vi "Process_day_file.vi"(2 "Filename":path=path "/G3_3 HD/EnFlo Data/Oct_2000/3_Oct") -> (6 "Day KW Hrs":dbl, 7 "Night KWHrs":dbl format="%.2f", 10 "Time":dbl)   [LabVIEW 2010]
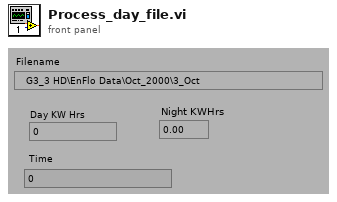
[diagram p1: front panel]
types:
  T1 = cluster{"second":i32, "minute":i32, "hour":i32, "day of month":i32, "month":i32, "year":i32, "day of week":i32, "day of year":i32, "is DST":i32}
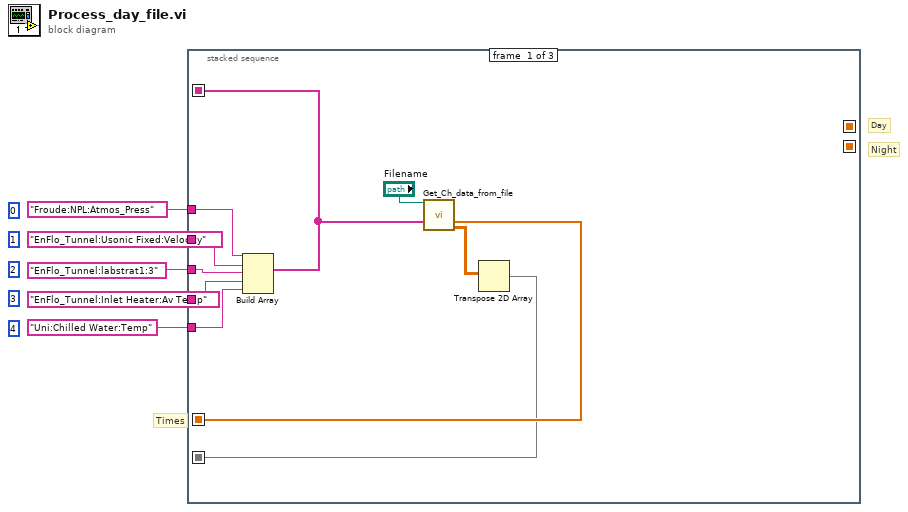
[diagram p0: block diagram]
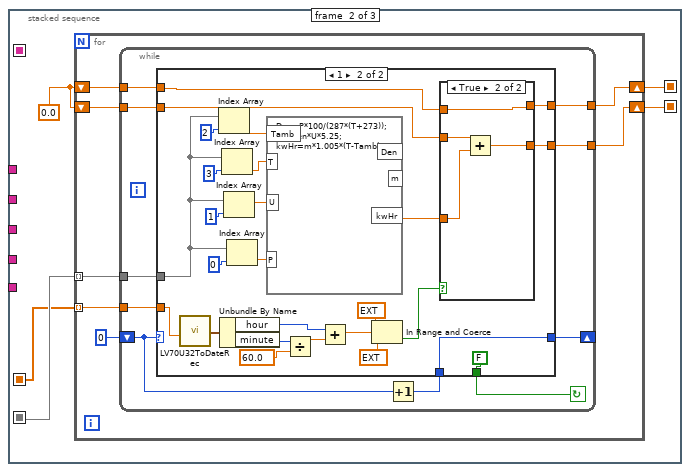
[diagram p2: hidden frame]
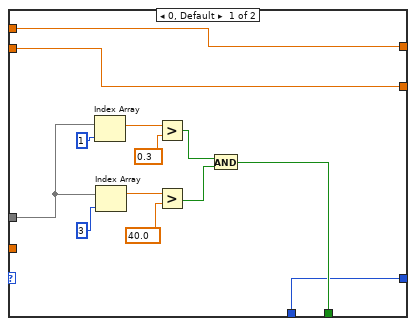
[diagram p3: hidden frame]
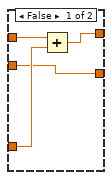
[diagram p4: hidden frame]
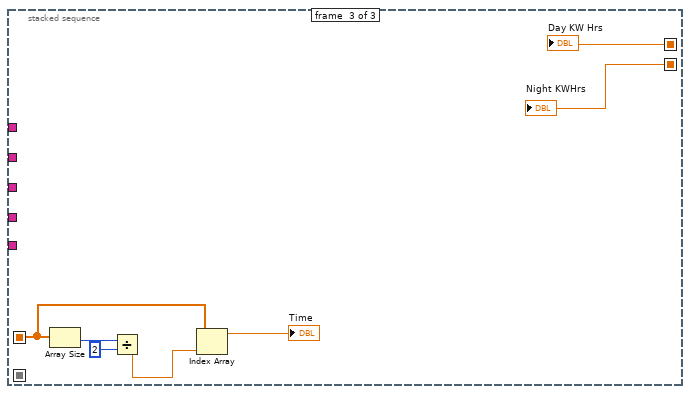
[diagram p5: hidden frame]
diagram:
  (unwired) 4
  (unwired) 3
  (unwired) 2
  (unwired) 1
  (unwired) 0
  # "Night"
  # "Day"
  # "Times"
  n1 = stacked-sequence {
    seq-local: [w9 _ _] -> [_ _ _]
    seq-local: [w8 _ _] -> [_ w18 w87]
    seq-local: [w6 _ _] -> [_ w20 _]
    seq-local: [_ w19 _] -> [_ _ w91]
    seq-local: [_ w16 _] -> [_ _ w85]
    tunnel: "Froude:NPL:Atmos_Press" -> [w15 _ _]
    tunnel: "EnFlo_Tunnel:Usonic Fixed:Velocity" -> [w14 _ _]
    tunnel: "EnFlo_Tunnel:labstrat1:3" -> [w13 _ _]
    tunnel: "EnFlo_Tunnel:Inlet Heater:Av Temp" -> [w12 _ _]
    tunnel: "Uni:Chilled Water:Temp" -> [w11 _ _]
    frame #0 {
      n2 = Build Array(w15, w14, w13, w12, w11) -> (w9:string[])
      n3 = call "Get_Ch_data_from_file.vi"("Filename"="Filename", "Channel names"=w9) -> ("Times"=w8:dbl[], "Ch Data"=w7:dbl[][])  [unwired: 2 in, 10 out]
      n4 = Transpose 2D Array(2D array=w7) -> (transposed array=w6:dbl[][])
    }
    frame #1 {
      w17 = 0.0
      n5 = for {
        tunnel: w20 -> [w26] mode=indexing
        shift-right: [w25] -> w19
        shift-left: w17 -> [w24]
        shift-right: [w21] -> w16
        shift-left: w17 -> [w22]
        tunnel: w18 -> [w23] mode=indexing
        n6 = while {
          tunnel: [w28] -> w21
          tunnel: w22 -> [w29]
          tunnel: w23 -> [w30]
          tunnel: w24 -> [w31]
          tunnel: [w32] -> w25
          tunnel: w26 -> [w37]
          shift-left: 0 -> [w35]
          shift-right: [w33] -> _
          stop <- w36 continue-if-true
          n7 = Increment(x=w35) -> (x+1=w34:i32)
          n8 = case shown="1" w35 {
            tunnel: w37 -> [w46 w72]
            tunnel: [w41 FALSE] -> w36
            tunnel: w34 -> [w40 w63]
            tunnel: [w40 w63] -> w33
            tunnel: [w39 w65] -> w32
            tunnel: w31 -> [w39 w66]
            tunnel: w30 -> [_ w62]
            tunnel: w29 -> [w38 w57]
            tunnel: [w38 w56] -> w28
            frame 0, Default {
              n9 = Index Array(array=w46, index=1 ("Index")) -> (element=w45:dbl)
              n10 = Index Array(array=w46, index=3 ("Index")) -> (element=w49:dbl)
              n11 = Greater?(x=w45, y=0.3) -> (0:w42:bool)
              n12 = Greater?(x=w49, y=40.0) -> (0:w43:bool)
              n13 = And(x=w42, y=w43) -> (x .and. y?=w41:bool)
            }
            frame 1 {
              n14 = call <vilib>:"LV70U32ToDateRec.vi"("Time"=w62) -> ("date time rec"=w61:T1)
              n15 = Index Array(array=w72, index=2 ("Index")) -> (element=w68:dbl)
              n16 = Unbundle By Name(w61) -> ("hour"=w52:i32, "minute"=w55:i32)
              n17 = Index Array(array=w72, index=3 ("Index")) -> (element=w69:dbl)
              n18 = Index Array(array=w72, index=1 ("Index")) -> (element=w70:dbl)
              n19 = Index Array(array=w72, index=0 ("Index")) -> (element=w71:dbl)
              n20 = formula code="Den=P*100/(287*(T+273));\nm=Den*U*5.25;\nkwHr=m*1.005*(T-Tamb)/30;"("Tamb"=w68, "T"=w69, "U"=w70, "P"=w71) -> ("kwHr"=w67:dbl)  [unwired: 2 out]
              n21 = Divide(x=w55, y=60.0) -> (x/y=w53:dbl)
              n22 = Add(x=w52, y=w53) -> (x+y=w51:dbl)
              n23 = In Range and Coerce(upper limit=ext 7.5 ("hi"), x=w51, lower limit=ext 0.5 ("lo")) -> (In Range?=w58:bool)  [unwired: 1 out]
              n24 = case shown="True" w58 {
                tunnel: w67 -> [w80 w82]
                tunnel: w66 -> [w79 w84]
                tunnel: [w78 w84] -> w65
                tunnel: w57 -> [w77 w83]
                tunnel: [w77 w81] -> w56
                frame False {
                  n25 = Add(x=w79, y=w80) -> (x+y=w78:dbl)
                }
                frame True {
                  n26 = Add(x=w83, y=w82) -> (x+y=w81:dbl)
                }
              }
            }
          }
        }
      }
    }
    frame #2 {
      n27 = Array Size(array=w87) -> (size(s)=w90:i32)
      n28 = Divide(x=w90, y=2) -> (x/y=w88:dbl)
      n29 = Index Array(array=w87, index=w88) -> (element=→"Time":dbl)
      "Day KW Hrs" <- w91
      "Night KWHrs" <- w85
    }
  }
